vi "Server.vi"() -> ()   [LabVIEW 2019]
uses:
  padrao_todos_os_dados_ENTRADA.ctl
  padrao_UCM.004.EEL.0300_ENTRADA.ctl
  padrao_UCM.004.EEL.0200_ENTRADA.ctl
  padrao_INTERNO.ctl
  padrao_todos_os_dados_SAIDA.ctl
  padrao_UCM.004.EEL.0300_SAIDA.ctl
  padrao_UCM.004.EEL.0200_SAIDA.ctl
  padrao_tipo_dado.ctl
  padrao_enum.ctl
  padrao_dados_cliente_para_server.ctl
  padrao_informacoes_meu_computador.ctl
  padrao_TAGS_prioridades_client.ctl
panel:
  in  "Help Button":bool
  in  "Abrir central de certificados":bool
  in  "Abre conversao e link":bool
  out "Array tipo de dado":T1[](array[typedef]) items=["Engenharia", "Puro(mA)"]
  in  "puro_todos_os_dados_ENTRADA":T2
  out "todos_dados_SAIDA":T6
  in  "engenharia_todos_os_dados_ENTRADA":T2
  in  "Editor Vinculos":bool
  in  "Calibração":bool
  in  "Closed":refnum<k5>
  out "IPs Conectados":string[](array[string])
  out "led_indica_server_ligado":bool
  out "status":string
  out "Clients Conectados":string[](array[string])
  out "Quantidade de Clients":i32
  out "Erro Nessa VI":errorcluster
  in  "[ESC]":bool
  # "SERVER"
  # "1)  Rode o Server antes de rodar os Clients\n2) Rode o Server: Aperte Ctrl+R ou rode na seta la em cima \n3) Verifique se o Led Acendeu:  Ele deve ficar laranja\n4) A cada Client ligado, ira aparecer na lista de clients\n5) Monitore a barra de status para saber o que está acontecendo\n6) Caso haja problema com troca de dados, utilize o debug ou monitore os dados.\n7) Para desligar o Server, desligue os Clients primeiro, quando a quantidade de Clients for igual a zero, aperte ESC ou no botão STOP."
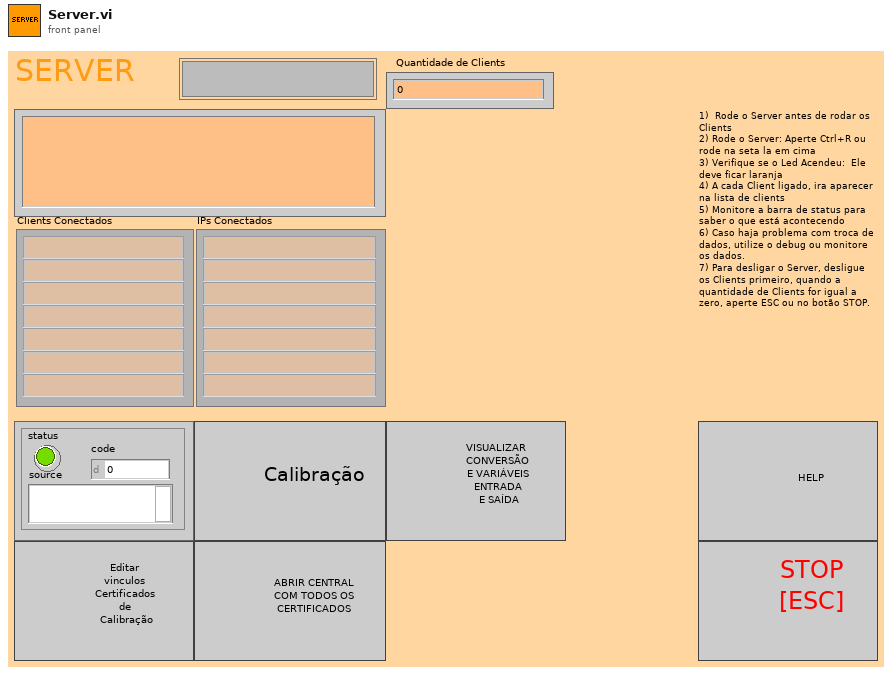
[diagram p1: front panel]
types:
  T1 = typedef "padrao_tipo_dado.ctl" = u16
  T2 = typedef "padrao_todos_os_dados_ENTRADA.ctl" = cluster{"UCM.004.EEL.0300_ENTRADA":T3, "UCM.004.EEL.0200_ENTRADA":T4, "INTERNO":T5}
  T3 = typedef "padrao_UCM.004.EEL.0300_ENTRADA.ctl" = cluster{"DIGITAL":cluster{"X30 1":bool, "X30 2":bool, "X30 3":bool, "X30 4":bool, "X30 5":bool, "X30 6":bool, "X30 7":bool, "X30 8":bool, "X30 9":bool, "X30 10":bool, "X30 11":bool, "X30 12":bool, "X30 13":bool, "X30 14":bool, "X30 15":bool, "X30 16":bool, "SPK-RD-ALR":bool, "SPK-RD-VVT":bool, "SPK-RD-FLL":bool, "SPW-RD-ALR":bool, "SPW-RD-VVT":bool, "SPW-RD-FLL":bool}, "ANALOGICO":cluster{"SKM-PA-BAR":i16, "SKM-PA-TQ":i16, "SKM-TI-TQ":i16, "SKM-PA-LAM":i16, "SKM-TI-LAM":i16, "SKM-PD-LAM":i16, "SKM-TI-WF":i16, "SKM-FIM-WF":i16, "SIT-PI-001":i16, "SKI-PD-ST":i16, "SIT-PI-MS1":i16, "SIT-PI-MS2":i16, "SKM-TI-KF":i16, "SPW-PD-P":i16, "SPK-PD-P":i16, "X32 16 ":i16, "X32 17":i16, "X32 18":i16, "X32 19":i16, "X32 20":i16, "X32 21":i16, "X32 22":i16, "X32 23":i16, "X32 24":i16, "SPK-RD-ST":i32, "SPW-RD-ST":i32, "SPK-RD-VEL":i32, "SPW-RD-VEL":i32, "SPK-RD-IA":i32, "SPW-RD-IA":i32, "SPK-RD-TU":i32, "SPW-RD-TU":i32, "SKM-TI-COR-KF":dbl, "SKM-DEN-COR-KF":dbl, "SKM-FIC-COR-KF":dbl, "SKM-TI-COR-AR":dbl, "SKM-DEN-COR-AR":dbl, "SPK-RD-CRT":dbl, "SPW-RD-CRT":dbl, "SKM-FIC-COR-AR":dbl}}
  T4 = typedef "padrao_UCM.004.EEL.0200_ENTRADA.ctl" = cluster{"DIGITAL":cluster{"SKS-LAH-S":bool, "SKS-LAH-W":bool, "SKS-LAH-K":bool, "SKS-MIN-W":bool, "SKS-MAX-W":bool, "SKS-MIN-K":bool, "SKS-MAX-K":bool, "X30-8":bool, "X30-9":bool, "X30-10":bool, "X30-11":bool, "X30-12":bool, "X30-13":bool, "X30-14":bool, "X30-15":bool, "X30-16":bool}, "ANALOGICO":cluster{"SKS-LC-K":i16, "SKS-LC-W":i16, "SHD-TI-AMB":i16, "X32-4":i16, "SHD-PI-01":i16, "SHD-PI-02":i16, "SIT-PI-MS3":i16, "SIT-PI-03":i16}}
  T5 = typedef "padrao_INTERNO.ctl" = cluster{"DIGITAL":cluster{"INTERNO-SI-SS-1":bool, "INTERNO-SI-SS-2":bool, "INTERNO-SI-SS-3":bool, "INTERNO-SS-SW-1":bool, "INTERNO-SS-SK-1":bool}, "ANALOGICO":cluster{"com_pc_analog":dbl}}
  T6 = typedef "padrao_todos_os_dados_SAIDA.ctl" = cluster{"UCM.004.EEL.0300_SAIDA":T7, "UCM.004.EEL.0200_SAIDA":T8, "INTERNO":T5}
  T7 = typedef "padrao_UCM.004.EEL.0300_SAIDA.ctl" = cluster{"DIGITAL":cluster{"SPK-CV-001":bool, "SPK-CV-002":bool, "SPK-CV-003":bool, "SPK-CV-004":bool, "SPK-CV-005":bool, "SPK-CV-006":bool, "SPK-CV-007":bool, "SPK-CV-008":bool, "SPW-CV-001":bool, "SPW-CV-002":bool, "SPW-CV-003":bool, "SPW-CV-004":bool, "SPW-CV-005":bool, "SPW-CV-006":bool, "SPW-CV-007":bool, "SPW-CV-008":bool, "SKM-CV-LAM":bool, "SKM-CV-COR":bool, "SKM-CV-JMP":bool, "SKI-CV-AR":bool, "SKI-CV-KF-ST":bool, "SKI-CV-KF-BY1":bool, "SKI-CV-WF-ST":bool, "SKI-CV-WF-BY1":bool, "SKI-CV-ST":bool, "SKI-CV-BY2":bool, "X31-27":bool, "X31-28":bool, "X31-29":bool, "X31-30":bool, "X31-31":bool, "X31-32":bool, "PID-PC-TQ-ON":bool, "PID-FC-AR-ON":bool, "PID-WF-ON":bool, "PID-KF-ON":bool, "PID-SA-WF-INV":bool, "PID-SA-KF-INV":bool, "PID-SA-AR-COR":bool, "SPK-WR-ON":bool, "SPW-WR-ON":bool, "SPK-WR-OFF":bool, "SPW-WR-OFF":bool}, "ANALOGICO":cluster{"SKM-PC-TQ":i16, "SKM-FC-AR":i16, "SKM-FC-WF":i16, "SKM-FC-KF":i16, "X33 5":i16, "X33 6":i16, "X33 7":i16, "X33 8":i16, "X33 9":i16, "X33 10":i16, "X33 11":i16, "X33 12":i16, "X33 13":i16, "X33 14":i16, "PID-PC-TQ-SP":i16, "PID-FC-AR-SP":i16, "PID-FC-WF-SP":i16, "PID-FC-KF-SP":i16, "PID-INC-WF-SP":i16, "PID-INC-KF-SP":i16, "SPK-WR-VEL":i32, "SPW-WR-VEL":i32, "SKM-FIC-COR-AR-MAX":dbl, "SKM-FIC-COR-AR-MIN":dbl, "SKM-FIC-COR-KF-MAX":dbl, "SKM-FIC-COR-KF-MIN":dbl, "PID-PC-TQ-GP":dbl, "PID-PC-TQ-GI":dbl, "PID-PC-TQ-GD":dbl, "PID-FC-AR-GP":dbl, "PID-FC-AR-GI":dbl, "PID-FC-AR-GD":dbl, "PID-FC-WF-GP":dbl, "PID-FC-WF-GI":dbl, "PID-FC-WF-GD":dbl, "PID-FC-KF-GP":dbl, "PID-FC-KF-GI":dbl, "PID-FC-KF-GD":dbl, "PID-INV-WF-GP":dbl, "PID-INV-WF-GI":dbl, "PID-INV-WF-GD":dbl, "PID-INV-KF-GP":dbl, "PID-INV-KF-GI":dbl, "PID-INV-KF-GD":dbl}}
  T8 = typedef "padrao_UCM.004.EEL.0200_SAIDA.ctl" = cluster{"DIGITAL":cluster{"SKS-CV-001":bool, "SKS-CV-002":bool, "SKS-CV-003":bool, "SKS-CV-004":bool, "SKS-CV-005":bool, "SKS-CV-006":bool, "SHD-CV-001":bool, "SHD-CV-002":bool, "SHD-ON-OFF":bool, "X31-10":bool, "X31-11":bool, "X31-12":bool, "X31-13":bool, "X31-14":bool, "X31-15":bool, "X31-16":bool}, "ANALOGICO":cluster{"GD-ST-ES":i16, "X33-2":i16}}
  T9 = typedef "padrao_enum.ctl" = enum16{"open-conection ", "data", "check-status", "Inicio"}
  T10 = enum32{"Invalid", "Standard", "Closed", "Hidden", "Minimized", "Maximized"}
  T11 = typedef "padrao_dados_cliente_para_server.ctl" = cluster{"todos_os_dados_saida":T6, "informacoes_meu_PC":T12, "padrao_prioridade_TAGs":T13}
  T12 = typedef "padrao_informacoes_meu_computador.ctl" = cluster{"Nome_computador":string, "IP_meu_computador":string, "Tipo de Dado":T1}
  T13 = typedef "padrao_TAGS_prioridades_client.ctl" = cluster{"TAG":string, "Tenho\nPrioridade?":bool}[]
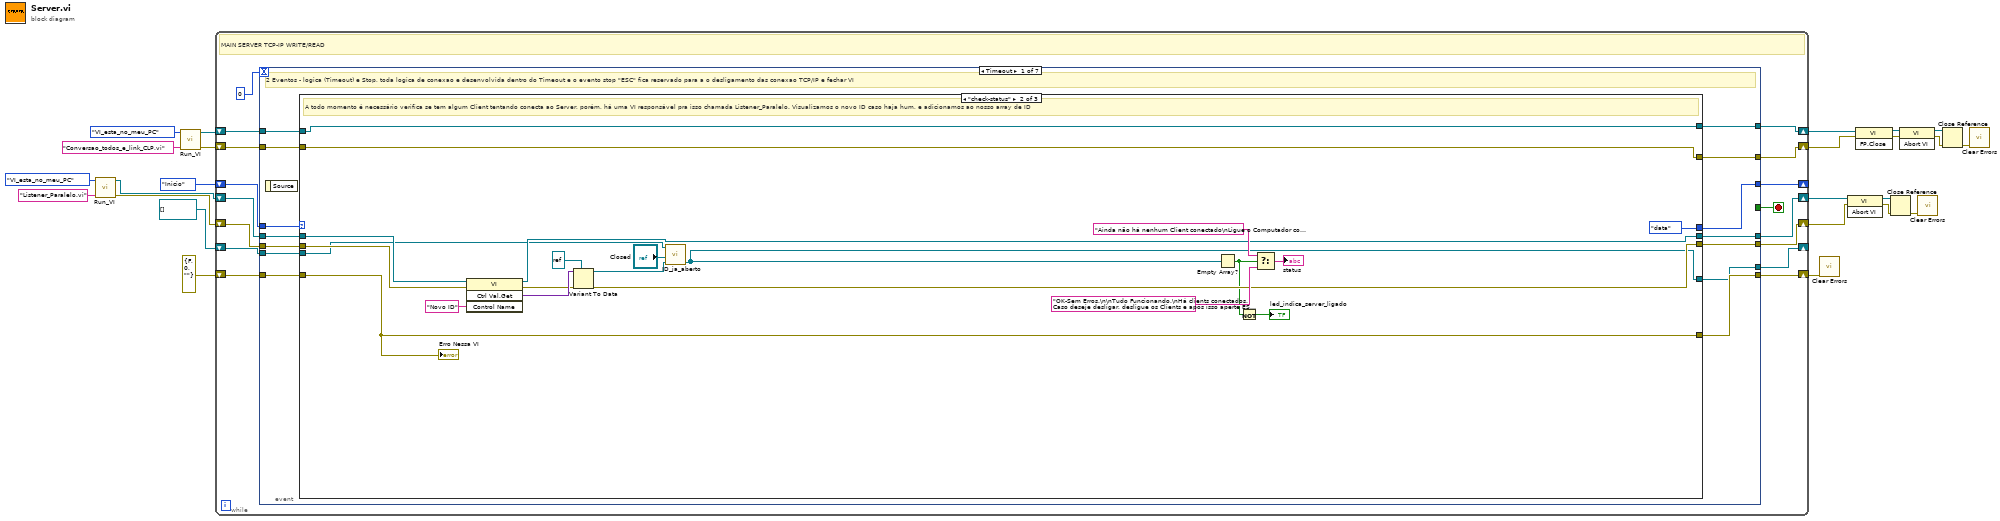
[diagram p0: block diagram]
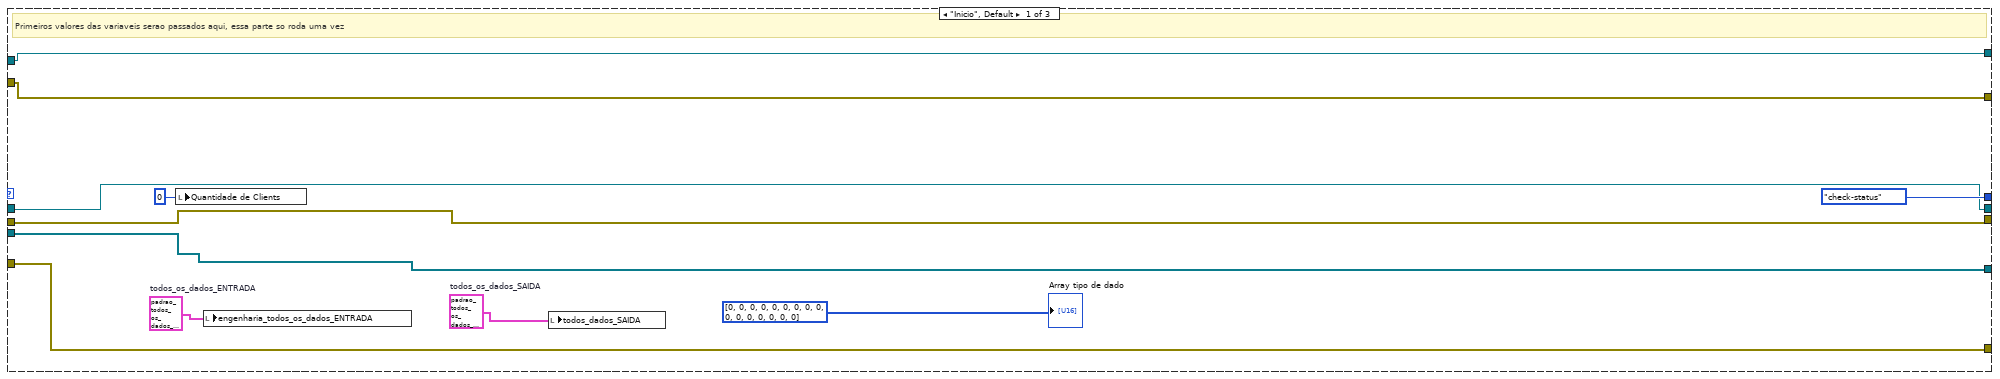
[diagram p2: hidden frame]
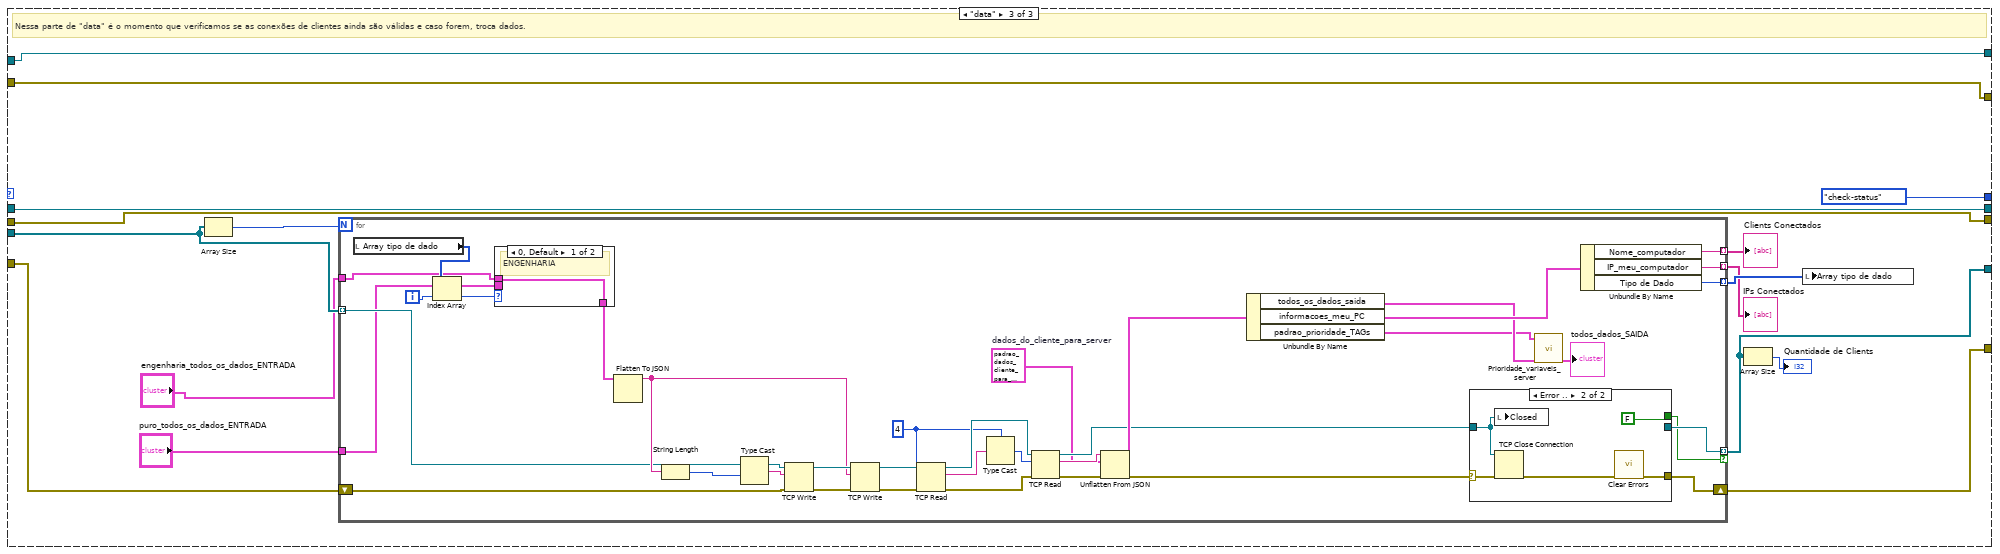
[diagram p3: hidden frame]
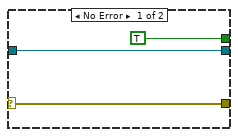
[diagram p5: hidden frame]
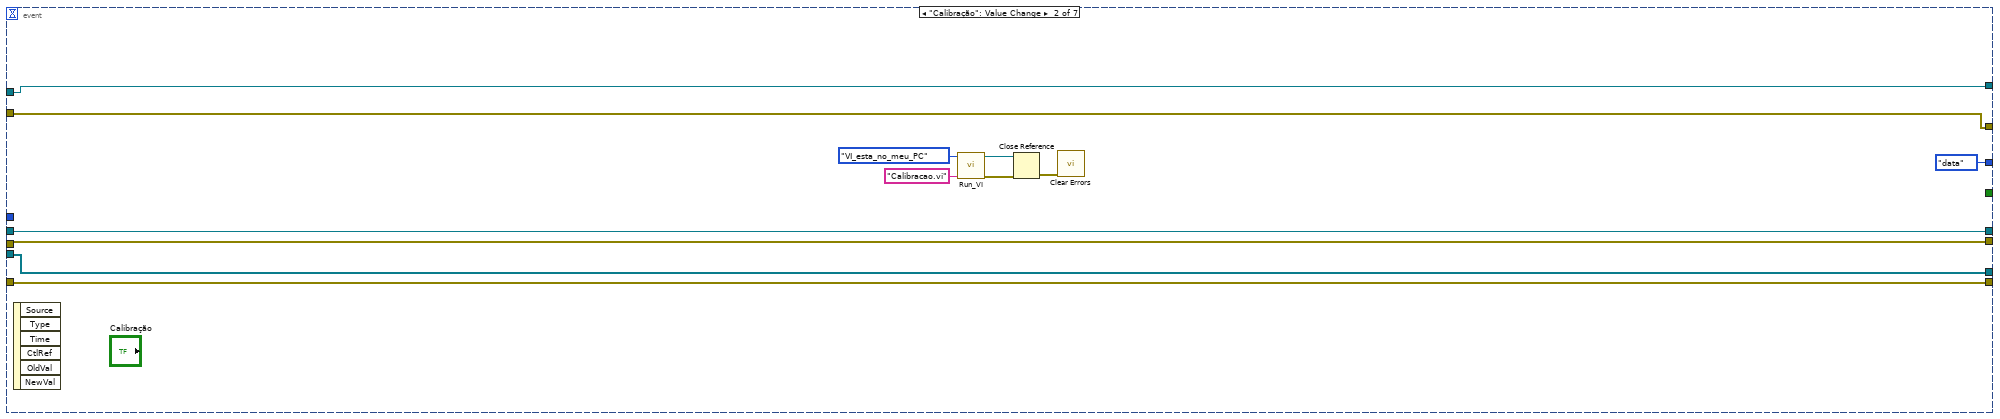
[diagram p6: hidden frame]
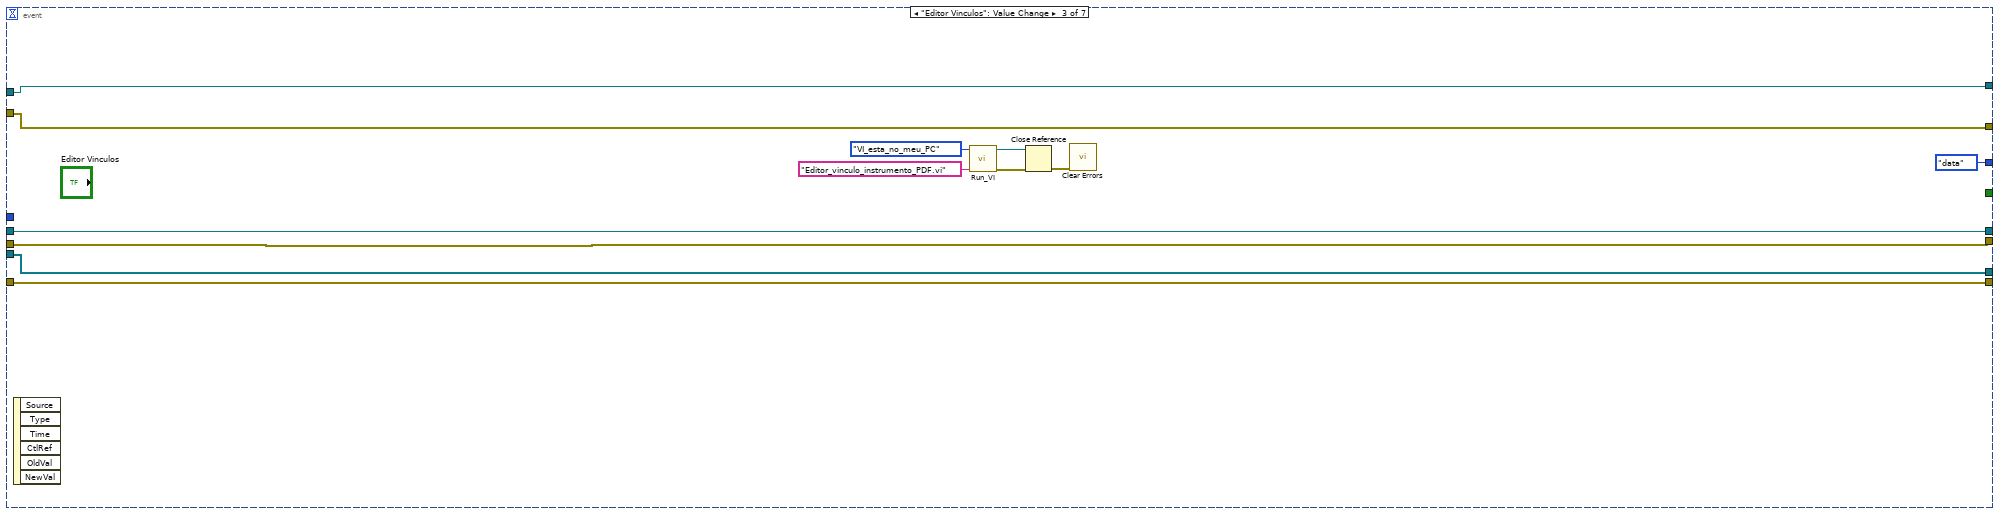
[diagram p7: hidden frame]
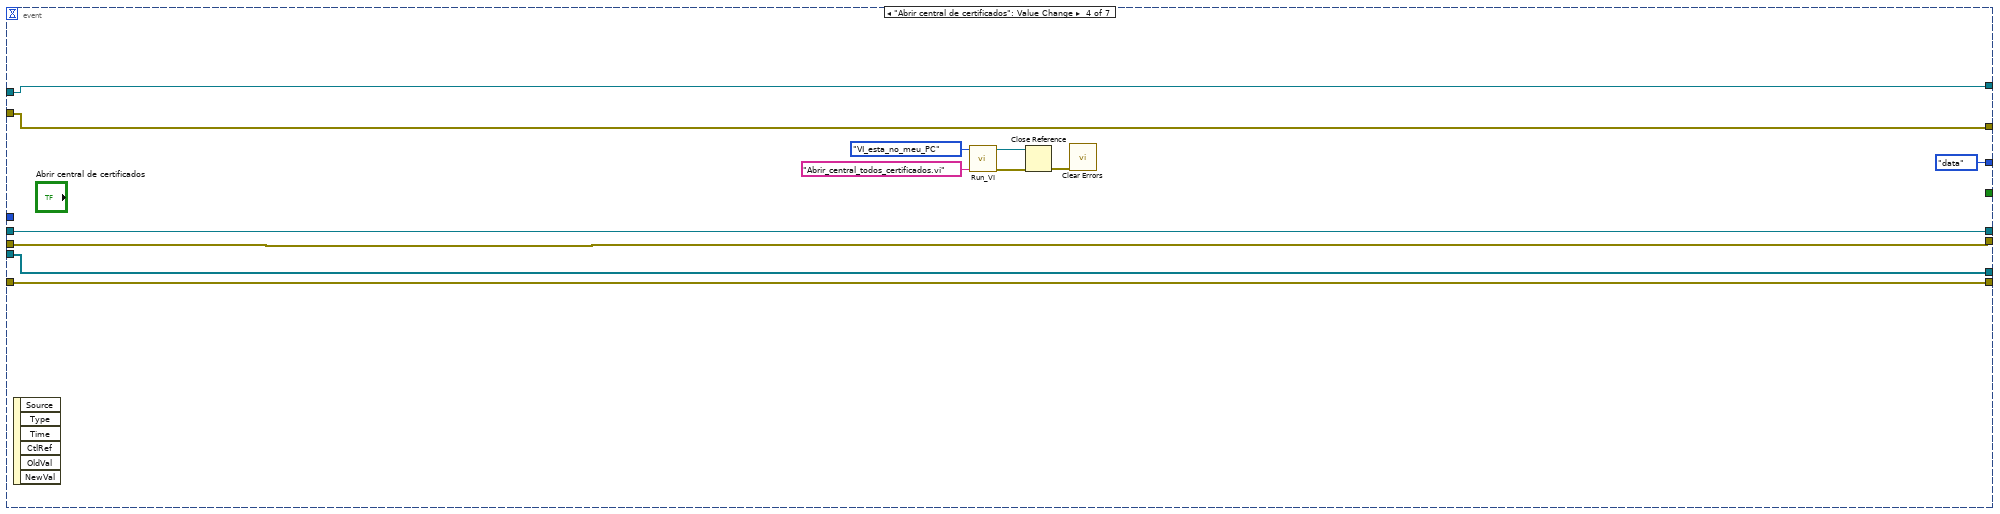
[diagram p8: hidden frame]
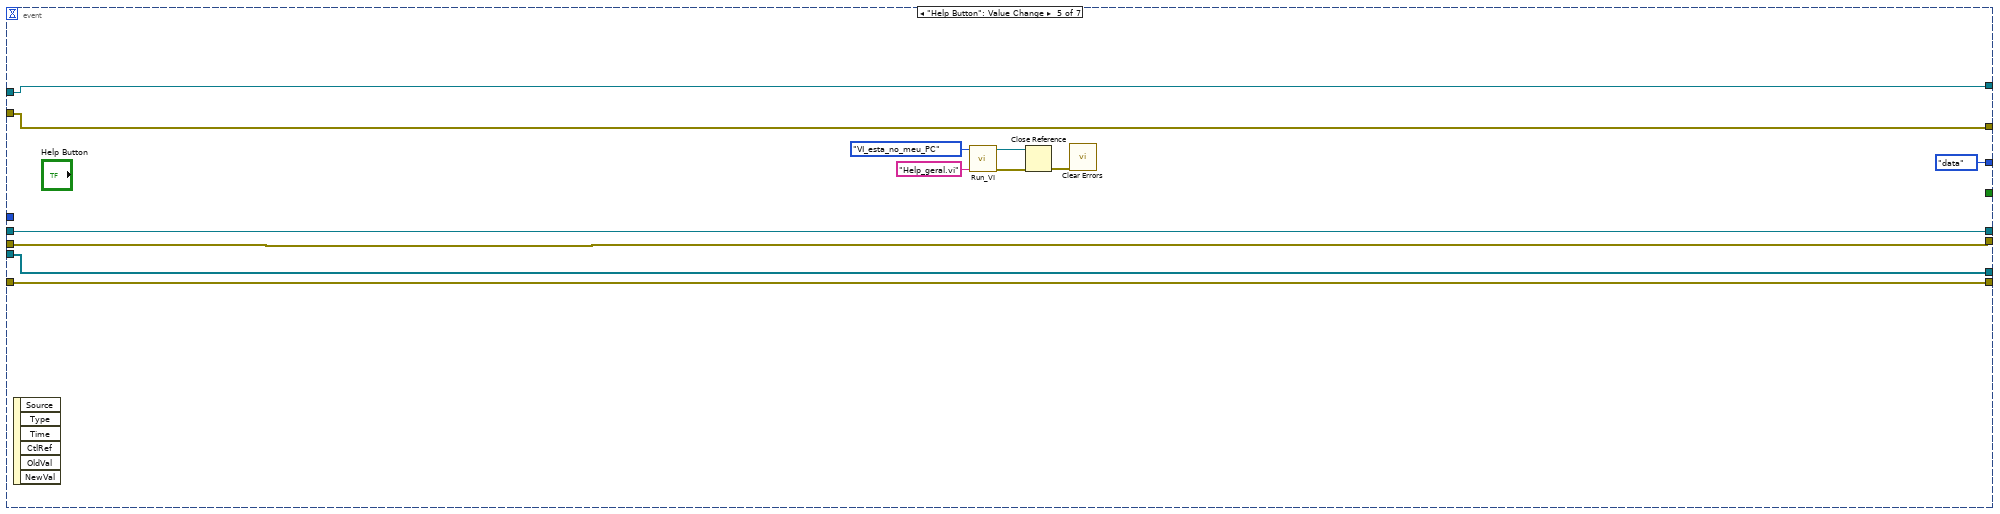
[diagram p9: hidden frame]
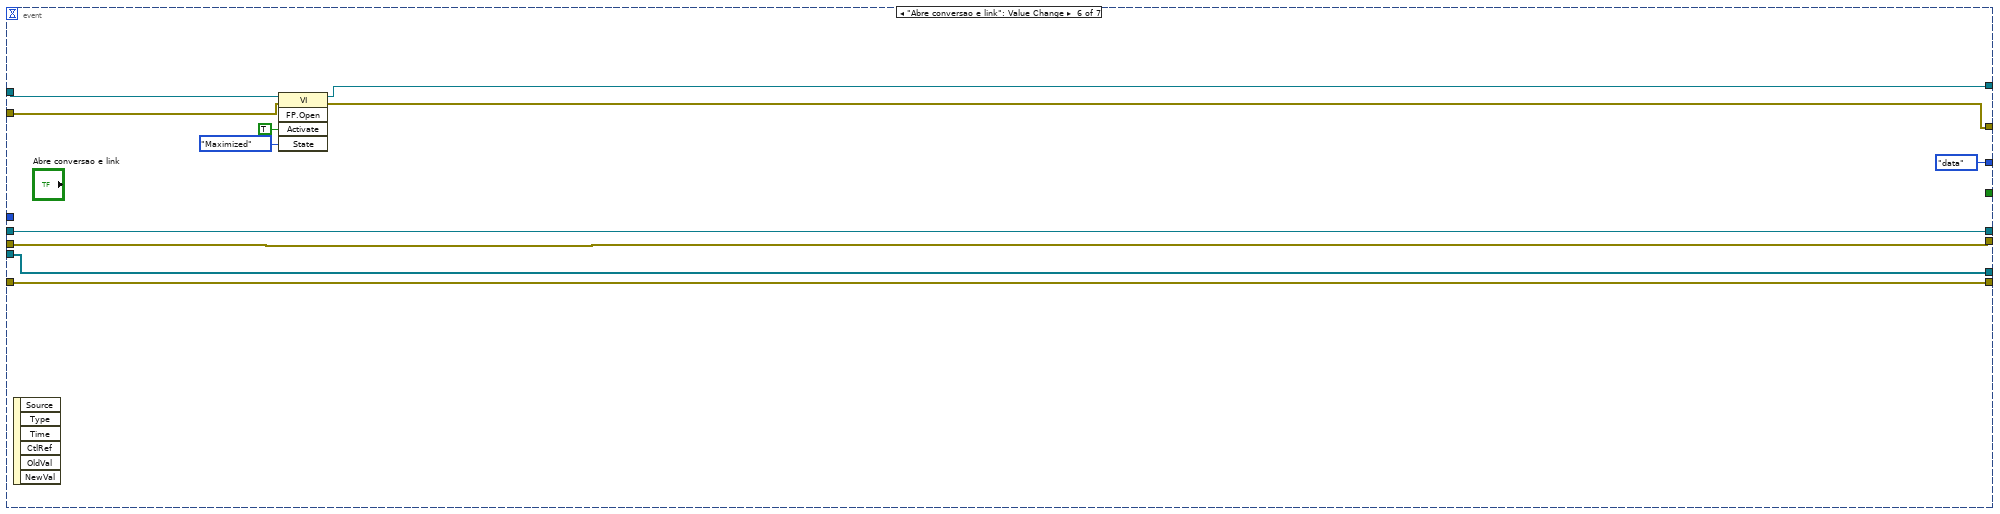
[diagram p10: hidden frame]
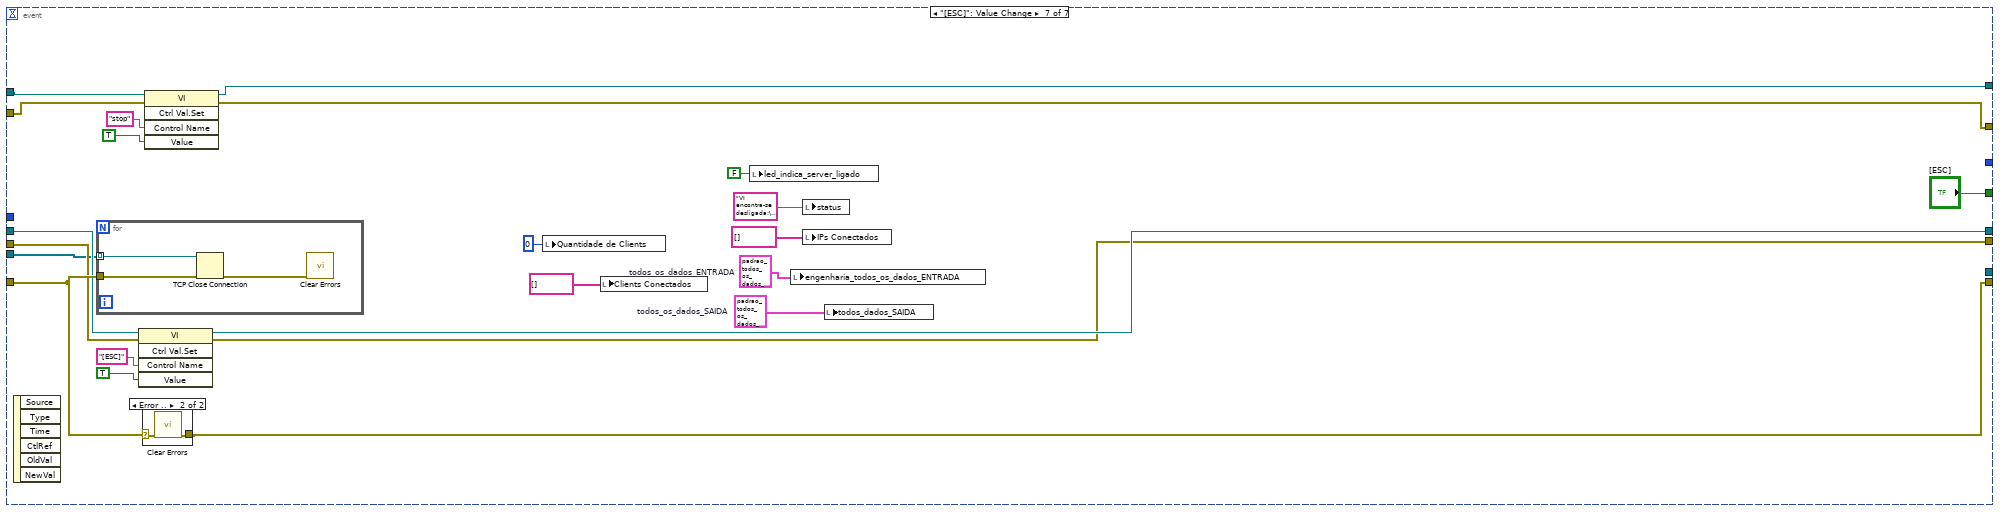
[diagram p11: hidden frame]
diagram:
  n1 = call "Run_VI.vi"("Nome.vi"="Listener_Paralelo.vi", "Origem_VI"=enum16{"VI_esta_no_meu_PC", "VI_esta_na_rede"}."VI_esta_no_meu_PC") -> ("error out"=w22:errorcluster, "reference out"=w21:refnum<vi>)  [unwired: 8 in]
  n2 = call "Run_VI.vi"("Nome.vi"="Conversao_todos_e_link_CLP.vi", "Origem_VI"=enum16{"VI_esta_no_meu_PC", "VI_esta_na_rede"}."VI_esta_no_meu_PC") -> ("error out"=w8:errorcluster, "reference out"=w9:refnum<vi>)  [unwired: 8 in]
  n3 = while {
    shift-right: [w34] -> _
    shift-left: padrao_enum."Inicio" ("Enum") -> [w39]
    shift-right: [w37] -> w13
    shift-left: errorcluster {"status"=FALSE, "code"=0, "source"=""} ("error constant") -> [w38]
    shift-right: [w33] -> _
    shift-left: refnum<k5>[] [] ("appended array") -> [w36]
    shift-right: [w30] -> w19
    shift-left: w21 -> [w32]
    shift-right: [w29] -> w18
    shift-left: w22 -> [w31]
    shift-right: [w26] -> w4
    shift-left: w9 -> [w28]
    shift-right: [w25] -> w3
    shift-left: w8 -> [w27]
    stop <- w40 stop-if-true
    # "MAIN SERVER TCP-IP WRITE/READ"
    n4 = event shown="[0] Timeout" {
      selector: _ -> [_ _ _ _ _ _ _]
      dyn-events: _ -> [_ _ _ _ _ _ _]
      timeout: 0 -> [_ _ _ _ _ _ _]
      tunnel: [_ _ _ _ _ _ "[ESC]"] -> w40
      tunnel: w39 -> [w51 _ _ _ _ _ _]
      tunnel: w38 -> [w54 w149 w161 w173 w185 w203 w228]
      tunnel: [w53 w149 w161 w173 w185 w203 w229] -> w37
      tunnel: w36 -> [w52 w150 w162 w174 w186 w204 w219]
      tunnel: [w50 padrao_enum."data" ("Enum") padrao_enum."data" ("Enum") padrao_enum."data" ("Enum") padrao_enum."data" ("Enum") padrao_enum."data" ("Enum") _] -> w34
      tunnel: [w49 w150 w162 w174 w186 w204 _] -> w33
      tunnel: w32 -> [w48 w152 w164 w176 w188 w206 w225]
      tunnel: w31 -> [w47 w151 w163 w175 w187 w205 w224]
      tunnel: [w46 w152 w164 w176 w188 w206 w221] -> w30
      tunnel: [w45 w151 w163 w175 w187 w205 w220] -> w29
      tunnel: w28 -> [w44 w154 w167 w179 w191 w202 w211]
      tunnel: w27 -> [w43 w153 w166 w178 w190 w201 w210]
      tunnel: [w42 w154 w167 w179 w191 w199 w209] -> w26
      tunnel: [w41 w153 w166 w178 w190 w198 w208] -> w25
      event Timeout {
        # "2 Eventos - logica (Timeout) e Stop, toda logica de conexao e desenvolvida dentro do Timeout e o evento stop \"ESC\" fica reservado para a o desligamento das conexao TCP/IP e fechar VI"
        n5 = event-data() -> ()  [unwired: 1 in, 1 out]
        n6 = case shown="\"check-status\"" w51 {
          tunnel: w54 -> [w64 w83 w101]
          tunnel: [w64 w83 w100] -> w53
          tunnel: w52 -> [w63 w73 w95]
          tunnel: [padrao_enum."check-status" ("Enum") padrao_enum."data" ("Enum") padrao_enum."check-status" ("Enum")] -> w50
          tunnel: [w63 w70 w94] -> w49
          tunnel: w48 -> [w61 w77 w99]
          tunnel: w47 -> [w60 w76 w98]
          tunnel: [w61 w75 w99] -> w46
          tunnel: [w60 w74 w98] -> w45
          tunnel: w44 -> [w57 w67 w88]
          tunnel: w43 -> [w56 w66 w87]
          tunnel: [w57 w67 w88] -> w42
          tunnel: [w56 w66 w87] -> w41
          frame "Inicio", Default {
            w58 = T6 {"UCM.004.EEL.0300_SAIDA"={"DIGITAL"={"SPK-CV-001"=FALSE, "SPK-CV-002"=FALSE, "SPK-CV-003"=FALSE, "SPK-CV-004"=FALSE, "SPK-CV-005"=FALSE, "SPK-CV-006"=FALSE, "SPK-CV-007"=FALSE, "SPK-CV-008"=FALSE, "SPW-CV-001"=FALSE, "SPW-CV-002"=FALSE, "SPW-CV-003"=FALSE, "SPW-CV-004"=FALSE, "SPW-CV-005"=FALSE, "SPW-CV-006"=FALSE, "SPW-CV-007"=FALSE, "SPW-CV-008"=FALSE, "SKM-CV-LAM"=FALSE, "SKM-CV-COR"=FALSE, "SKM-CV-JMP"=FALSE, "SKI-CV-AR"=FALSE, "SKI-CV-KF-ST"=FALSE, "SKI-CV-KF-BY1"=FALSE, "SKI-CV-WF-ST"=FALSE, "SKI-CV-WF-BY1"=FALSE, "SKI-CV-ST"=FALSE, "SKI-CV-BY2"=FALSE, "X31-27"=FALSE, "X31-28"=FALSE, "X31-29"=FALSE, "X31-30"=FALSE, "X31-31"=FALSE, "X31-32"=FALSE, "PID-PC-TQ-ON"=FALSE, "PID-FC-AR-ON"=FALSE, "PID-WF-ON"=FALSE, "PID-KF-ON"=FALSE, "PID-SA-WF-INV"=FALSE, "PID-SA-KF-INV"=FALSE, "PID-SA-AR-COR"=FALSE, "SPK-WR-ON"=FALSE, "SPW-WR-ON"=FALSE, "SPK-WR-OFF"=FALSE, "SPW-WR-OFF"=FALSE}, "ANALOGICO"={"SKM-PC-TQ"=0, "SKM-FC-AR"=0, "SKM-FC-WF"=0, "SKM-FC-KF"=0, "X33 5"=0, "X33 6"=0, "X33 7"=0, "X33 8"=0, "X33 9"=0, "X33 10"=0, "X33 11"=0, "X33 12"=0, "X33 13"=0, "X33 14"=0, "PID-PC-TQ-SP"=0, "PID-FC-AR-SP"=0, "PID-FC-WF-SP"=0, "PID-FC-KF-SP"=0, "PID-INC-WF-SP"=0, "PID-INC-KF-SP"=0, "SPK-WR-VEL"=0, "SPW-WR-VEL"=0, "SKM-FIC-COR-AR-MAX"=0.0, "SKM-FIC-COR-AR-MIN"=0.0, "SKM-FIC-COR-KF-MAX"=0.0, "SKM-FIC-COR-KF-MIN"=0.0, "PID-PC-TQ-GP"=0.0, "PID-PC-TQ-GI"=0.0, "PID-PC-TQ-GD"=0.0, "PID-FC-AR-GP"=0.0, "PID-FC-AR-GI"=0.0, "PID-FC-AR-GD"=0.0, "PID-FC-WF-GP"=0.0, "PID-FC-WF-GI"=0.0, "PID-FC-WF-GD"=0.0, "PID-FC-KF-GP"=0.0, "PID-FC-KF-GI"=0.0, "PID-FC-KF-GD"=0.0, "PID-INV-WF-GP"=0.0, "PID-INV-WF-GI"=0.0, "PID-INV-WF-GD"=0.0, "PID-INV-KF-GP"=0.0, "PID-INV-KF-GI"=0.0, "PID-INV-KF-GD"=0.0}}, "UCM.004.EEL.0200_SAIDA"={"DIGITAL"={"SKS-CV-001"=FALSE, "SKS-CV-002"=FALSE, "SKS-CV-003"=FALSE, "SKS-CV-004"=FALSE, "SKS-CV-005"=FALSE, "SKS-CV-006"=FALSE, "SHD-CV-001"=FALSE, "SHD-CV-002"=FALSE, "SHD-ON-OFF"=FALSE, "X31-10"=FALSE, "X31-11"=FALSE, "X31-12"=FALSE, "X31-13"=FALSE, "X31-14"=FALSE, "X31-15"=FALSE, "X31-16"=FALSE}, "ANALOGICO"={"GD-ST-ES"=0, "X33-2"=0}}, "INTERNO"={"DIGITAL"={"INTERNO-SI-SS-1"=FALSE, "INTERNO-SI-SS-2"=FALSE, "INTERNO-SI-SS-3"=FALSE, "INTERNO-SS-SW-1"=FALSE, "INTERNO-SS-SK-1"=FALSE}, "ANALOGICO"={"com_pc_analog"=0.0}}}  # todos_os_dados_SAIDA
            w59 = T2 {"UCM.004.EEL.0300_ENTRADA"={"DIGITAL"={"X30 1"=FALSE, "X30 2"=FALSE, "X30 3"=FALSE, "X30 4"=FALSE, "X30 5"=FALSE, "X30 6"=FALSE, "X30 7"=FALSE, "X30 8"=FALSE, "X30 9"=FALSE, "X30 10"=FALSE, "X30 11"=FALSE, "X30 12"=FALSE, "X30 13"=FALSE, "X30 14"=FALSE, "X30 15"=FALSE, "X30 16"=FALSE, "SPK-RD-ALR"=FALSE, "SPK-RD-VVT"=FALSE, "SPK-RD-FLL"=FALSE, "SPW-RD-ALR"=FALSE, "SPW-RD-VVT"=FALSE, "SPW-RD-FLL"=FALSE}, "ANALOGICO"={"SKM-PA-BAR"=0, "SKM-PA-TQ"=0, "SKM-TI-TQ"=0, "SKM-PA-LAM"=0, "SKM-TI-LAM"=0, "SKM-PD-LAM"=0, "SKM-TI-WF"=0, "SKM-FIM-WF"=0, "SIT-PI-001"=0, "SKI-PD-ST"=0, "SIT-PI-MS1"=0, "SIT-PI-MS2"=0, "SKM-TI-KF"=0, "SPW-PD-P"=0, "SPK-PD-P"=0, "X32 16 "=0, "X32 17"=0, "X32 18"=0, "X32 19"=0, "X32 20"=0, "X32 21"=0, "X32 22"=0, "X32 23"=0, "X32 24"=0, "SPK-RD-ST"=0, "SPW-RD-ST"=0, "SPK-RD-VEL"=0, "SPW-RD-VEL"=0, "SPK-RD-IA"=0, "SPW-RD-IA"=0, "SPK-RD-TU"=0, "SPW-RD-TU"=0, "SKM-TI-COR-KF"=0.0, "SKM-DEN-COR-KF"=0.0, "SKM-FIC-COR-KF"=0.0, "SKM-TI-COR-AR"=0.0, "SKM-DEN-COR-AR"=0.0, "SPK-RD-CRT"=0.0, "SPW-RD-CRT"=0.0, "SKM-FIC-COR-AR"=0.0}}, "UCM.004.EEL.0200_ENTRADA"={"DIGITAL"={"SKS-LAH-S"=FALSE, "SKS-LAH-W"=FALSE, "SKS-LAH-K"=FALSE, "SKS-MIN-W"=FALSE, "SKS-MAX-W"=FALSE, "SKS-MIN-K"=FALSE, "SKS-MAX-K"=FALSE, "X30-8"=FALSE, "X30-9"=FALSE, "X30-10"=FALSE, "X30-11"=FALSE, "X30-12"=FALSE, "X30-13"=FALSE, "X30-14"=FALSE, "X30-15"=FALSE, "X30-16"=FALSE}, "ANALOGICO"={"SKS-LC-K"=0, "SKS-LC-W"=0, "SHD-TI-AMB"=0, "X32-4"=0, "SHD-PI-01"=0, "SHD-PI-02"=0, "SIT-PI-MS3"=0, "SIT-PI-03"=0}}, "INTERNO"={"DIGITAL"={"INTERNO-SI-SS-1"=FALSE, "INTERNO-SI-SS-2"=FALSE, "INTERNO-SI-SS-3"=FALSE, "INTERNO-SS-SW-1"=FALSE, "INTERNO-SS-SK-1"=FALSE}, "ANALOGICO"={"com_pc_analog"=0.0}}}  # todos_os_dados_ENTRADA
            w55 = T1[] [0, 0, 0, 0, 0, 0, 0, 0, 0, 0, 0, 0, 0, 0, 0, 0] items=["Engenharia", "Puro(mA)"] ("Array")
            # "Primeiros valores das variaveis serao passados aqui, essa parte so roda uma vez"
            n7 = local write "Quantidade de Clients"(0 ("size(s)")) -> ()
            n8 = local write "engenharia_todos_os_dados_ENTRADA"(w59) -> ()
            n9 = local write "todos_dados_SAIDA"(w58) -> ()
            "Array tipo de dado" <- w55
          }
          frame "check-status" {
            # "A todo momento é necessário verifica se tem algum Client tentando conecta ao Server, porém, há uma VI responsável pra isso chamada Listener_Paralelo. Visualizamos o novo ID caso haja hum, e adicionamos ao nosso array de ID"
            n10 = invoke class="VI" method="Ctrl Val.Get"(reference=w77, error in=w76, "Control Name"="Novo ID") -> (reference out=w75:refnum<vi>, error out=w78:errorcluster, "Get Control Value Variant"=w80:variant)  [unwired: 1 in, 1 out]
            n11 = Variant To Data(error in=w78, type=refnum<k5> refnum ("listener ID"), Variant=w80) -> (data=w71:refnum<k5>, error out=w74:errorcluster)
            n12 = call "ID_ja_aberto.vi"("Conexao nova"=w71, "Conexao fechada"="Closed", "Entrada Array Conexao"=w73) -> ("Saida Array Conexao"=w70:refnum<k5>[])  [unwired: 8 in]
            n13 = Empty Array?(array=w70) -> (empty?=w68:bool)
            n14 = Not(x=w68) -> (.not. x?=→"led_indica_server_ligado":bool)
            n15 = Select(t="Ainda não há nenhum Client conectado\nLigue o Computador com o Client que deseje utilizar\nAperte ESC caso deseje encerrar", s=w68, f="OK-Sem Erros.\n\nTudo Funcionando.\nHá clients conectados. Caso deseje desligar, desligue os Clients e após isso aperte ESC nessa VI") -> (s? t:f=→"status":string)
            "Erro Nessa VI" <- w83
          }
          frame "data" {
            # "Nessa parte de \"data\" é o momento que verificamos se as conexões de clientes ainda são válidas e caso forem, troca dados."
            n16 = Array Size(array=w95) -> (size(s)=w96:i32)
            n17 = for {
              N: w96 -> [_]
              tunnel: w95 -> [w132] mode=indexing
              shift-right: [w116] -> w100
              shift-left: w101 -> [w138]
              tunnel: [w118] -> w94 mode=indexing if=w117
              tunnel: [w121] -> w91 mode=indexing
              tunnel: [w120] -> w93 mode=indexing
              tunnel: [w119] -> w92 mode=indexing
              tunnel: "engenharia_todos_os_dados_ENTRADA" -> [w107]
              tunnel: "puro_todos_os_dados_ENTRADA" -> [w106]
              i -> [w112]
              w104 = T11 {"todos_os_dados_saida"={"UCM.004.EEL.0300_SAIDA"={"DIGITAL"={"SPK-CV-001"=FALSE, "SPK-CV-002"=FALSE, "SPK-CV-003"=FALSE, "SPK-CV-004"=FALSE, "SPK-CV-005"=FALSE, "SPK-CV-006"=FALSE, "SPK-CV-007"=FALSE, "SPK-CV-008"=FALSE, "SPW-CV-001"=FALSE, "SPW-CV-002"=FALSE, "SPW-CV-003"=FALSE, "SPW-CV-004"=FALSE, "SPW-CV-005"=FALSE, "SPW-CV-006"=FALSE, "SPW-CV-007"=FALSE, "SPW-CV-008"=FALSE, "SKM-CV-LAM"=FALSE, "SKM-CV-COR"=FALSE, "SKM-CV-JMP"=FALSE, "SKI-CV-AR"=FALSE, "SKI-CV-KF-ST"=FALSE, "SKI-CV-KF-BY1"=FALSE, "SKI-CV-WF-ST"=FALSE, "SKI-CV-WF-BY1"=FALSE, "SKI-CV-ST"=FALSE, "SKI-CV-BY2"=FALSE, "X31-27"=FALSE, "X31-28"=FALSE, "X31-29"=FALSE, "X31-30"=FALSE, "X31-31"=FALSE, "X31-32"=FALSE, "PID-PC-TQ-ON"=FALSE, "PID-FC-AR-ON"=FALSE, "PID-WF-ON"=FALSE, "PID-KF-ON"=FALSE, "PID-SA-WF-INV"=FALSE, "PID-SA-KF-INV"=FALSE, "PID-SA-AR-COR"=FALSE, "SPK-WR-ON"=FALSE, "SPW-WR-ON"=FALSE, "SPK-WR-OFF"=FALSE, "SPW-WR-OFF"=FALSE}, "ANALOGICO"={"SKM-PC-TQ"=0, "SKM-FC-AR"=0, "SKM-FC-WF"=0, "SKM-FC-KF"=0, "X33 5"=0, "X33 6"=0, "X33 7"=0, "X33 8"=0, "X33 9"=0, "X33 10"=0, "X33 11"=0, "X33 12"=0, "X33 13"=0, "X33 14"=0, "PID-PC-TQ-SP"=0, "PID-FC-AR-SP"=0, "PID-FC-WF-SP"=0, "PID-FC-KF-SP"=0, "PID-INC-WF-SP"=0, "PID-INC-KF-SP"=0, "SPK-WR-VEL"=0, "SPW-WR-VEL"=0, "SKM-FIC-COR-AR-MAX"=0.0, "SKM-FIC-COR-AR-MIN"=0.0, "SKM-FIC-COR-KF-MAX"=0.0, "SKM-FIC-COR-KF-MIN"=0.0, "PID-PC-TQ-GP"=0.0, "PID-PC-TQ-GI"=0.0, "PID-PC-TQ-GD"=0.0, "PID-FC-AR-GP"=0.0, "PID-FC-AR-GI"=0.0, "PID-FC-AR-GD"=0.0, "PID-FC-WF-GP"=0.0, "PID-FC-WF-GI"=0.0, "PID-FC-WF-GD"=0.0, "PID-FC-KF-GP"=0.0, "PID-FC-KF-GI"=0.0, "PID-FC-KF-GD"=0.0, "PID-INV-WF-GP"=0.0, "PID-INV-WF-GI"=0.0, "PID-INV-WF-GD"=0.0, "PID-INV-KF-GP"=0.0, "PID-INV-KF-GI"=0.0, "PID-INV-KF-GD"=0.0}}, "UCM.004.EEL.0200_SAIDA"={"DIGITAL"={"SKS-CV-001"=FALSE, "SKS-CV-002"=FALSE, "SKS-CV-003"=FALSE, "SKS-CV-004"=FALSE, "SKS-CV-005"=FALSE, "SKS-CV-006"=FALSE, "SHD-CV-001"=FALSE, "SHD-CV-002"=FALSE, "SHD-ON-OFF"=FALSE, "X31-10"=FALSE, "X31-11"=FALSE, "X31-12"=FALSE, "X31-13"=FALSE, "X31-14"=FALSE, "X31-15"=FALSE, "X31-16"=FALSE}, "ANALOGICO"={"GD-ST-ES"=0, "X33-2"=0}}, "INTERNO"={"DIGITAL"={"INTERNO-SI-SS-1"=FALSE, "INTERNO-SI-SS-2"=FALSE, "INTERNO-SI-SS-3"=FALSE, "INTERNO-SS-SW-1"=FALSE, "INTERNO-SS-SK-1"=FALSE}, "ANALOGICO"={"com_pc_analog"=0.0}}}, "informacoes_meu_PC"={"Nome_computador"="", "IP_meu_computador"="", "Tipo de Dado"=0}, "padrao_prioridade_TAGs"=[]}  # dados_do_cliente_para_server
              w125 = 4 ("bytes to read")
              n18 = local read "Array tipo de dado"() -> (w113:T1[])
              n19 = Index Array(array=w113, index=w112) -> (element=w108:T1)
              n20 = case shown="0, Default" w108 {
                tunnel: w107 -> [w139 _]
                tunnel: w106 -> [_ w140]
                tunnel: [w139 w140] -> w105
                frame 0, Default {
                  # "ENGENHARIA"
                }
                frame 1 {
                  # "PURO"
                }
              }
              n21 = Flatten To JSON(anything=w105) -> (JSON string=w133:string)  [unwired: 2 in, 1 out]
              n22 = String Length(string=w133) -> (length=w135:i32)
              n23 = Type Cast(x=w135) -> (*(type *) &x=w134:string)  [unwired: 1 in]
              n24 = TCP Write(connection ID=w132, data in=w134, error in (no error)=w138) -> (connection ID out=w136:refnum<k5>, error out=w137:errorcluster)  [unwired: 2 out]
              n25 = TCP Write(connection ID=w136, data in=w133, error in (no error)=w137) -> (connection ID out=w131:refnum<k5>, error out=w130:errorcluster)  [unwired: 2 out]
              n26 = TCP Read(connection ID=w131, bytes to read=w125, error in (no error)=w130) -> (connection ID out=w129:refnum<k5>, data out=w126:string, error out=w128:errorcluster)  [unwired: 2 in]
              n27 = Type Cast(type=w125, x=w126) -> (*(type *) &x=w124:i32)
              n28 = TCP Read(connection ID=w129, bytes to read=w124, error in (no error)=w128) -> (connection ID out=w115:refnum<k5>, data out=w123:string, error out=w127:errorcluster)  [unwired: 2 in]
              n29 = Unflatten From JSON(JSON string=w123, type and defaults=w104, error in (no error)=w127) -> (value=w122:T11, error out=w114:errorcluster)  [unwired: 4 in]
              n30 = Unbundle By Name(w122) -> ("todos_os_dados_saida"=w110:T6, "informacoes_meu_PC"=w111:T12, "padrao_prioridade_TAGs"=w109:T13)
              n31 = case shown="Error .." w114 {
                selector: w114 -> [w143 w145]
                tunnel: w115 -> [w141 w144]
                tunnel: [w143 w148] -> w116
                tunnel: [TRUE FALSE] -> w117
                tunnel: [w141 _] -> w118
                frame No Error {
                }
                frame Error {
                  n32 = local write "Closed"(w144) -> ()
                  n33 = TCP Close Connection(connection ID=w144, error in (no error)=w145) -> (error out=w146:errorcluster)  [unwired: 1 in, 1 out]
                  n34 = call <vilib>:"Clear Errors.vi"("error in (no error)"=w146) -> ("error out"=w148:errorcluster)  [unwired: 5 in, 1 out]
                }
              }
              n35 = call "Prioridade_variaveis_server.vi"("dados_entrada_vindo_client"=w110, "padrao_TAGS_prioridade_client"=w109) -> ("dados_entrada_para_clp_priorizado"=→"todos_dados_SAIDA":T6)  [unwired: 9 in]
              n36 = Unbundle By Name(w111) -> ("Nome_computador"=w121:string, "IP_meu_computador"=w119:string, "Tipo de Dado"=w120:T1)
            }
            "Clients Conectados" <- w91
            "IPs Conectados" <- w92
            n37 = Array Size(array=w94) -> (size(s)=→"Quantidade de Clients":i32)
            n38 = local write "Array tipo de dado"(w93) -> ()
          }
        }
      }
      event "Calibração": Value Change {
        n39 = event-data() -> ()  [unwired: 1 in, 6 out]
        n40 = call "Run_VI.vi"("Nome.vi"="Calibracao.vi", "Origem_VI"=enum16{"VI_esta_no_meu_PC", "VI_esta_na_rede"}."VI_esta_no_meu_PC") -> ("error out"=w158:errorcluster, "reference out"=w159:refnum<vi>)  [unwired: 8 in]
        n41 = Close Reference(reference=w159, error in (no error)=w158) -> (error out=w157:errorcluster)
        n42 = call <vilib>:"Clear Errors.vi"("error in (no error)"=w157) -> ()  [unwired: 5 in, 2 out]
      }
      event "Editor Vinculos": Value Change {
        n43 = event-data() -> ()  [unwired: 1 in, 6 out]
        n44 = call "Run_VI.vi"("Nome.vi"="Editor_vinculo_instrumento_PDF.vi", "Origem_VI"=enum16{"VI_esta_no_meu_PC", "VI_esta_na_rede"}."VI_esta_no_meu_PC") -> ("error out"=w170:errorcluster, "reference out"=w171:refnum<vi>)  [unwired: 8 in]
        n45 = Close Reference(reference=w171, error in (no error)=w170) -> (error out=w169:errorcluster)
        n46 = call <vilib>:"Clear Errors.vi"("error in (no error)"=w169) -> ()  [unwired: 5 in, 2 out]
      }
      event "Abrir central de certificados": Value Change {
        n47 = event-data() -> ()  [unwired: 1 in, 6 out]
        n48 = call "Run_VI.vi"("Nome.vi"="Abrir_central_todos_certificados.vi", "Origem_VI"=enum16{"VI_esta_no_meu_PC", "VI_esta_na_rede"}."VI_esta_no_meu_PC") -> ("error out"=w182:errorcluster, "reference out"=w183:refnum<vi>)  [unwired: 8 in]
        n49 = Close Reference(reference=w183, error in (no error)=w182) -> (error out=w181:errorcluster)
        n50 = call <vilib>:"Clear Errors.vi"("error in (no error)"=w181) -> ()  [unwired: 5 in, 2 out]
      }
      event "Help Button": Value Change {
        n51 = event-data() -> ()  [unwired: 1 in, 6 out]
        n52 = call "Run_VI.vi"("Nome.vi"="Help_geral.vi", "Origem_VI"=enum16{"VI_esta_no_meu_PC", "VI_esta_na_rede"}."VI_esta_no_meu_PC") -> ("error out"=w194:errorcluster, "reference out"=w195:refnum<vi>)  [unwired: 8 in]
        n53 = Close Reference(reference=w195, error in (no error)=w194) -> (error out=w193:errorcluster)
        n54 = call <vilib>:"Clear Errors.vi"("error in (no error)"=w193) -> ()  [unwired: 5 in, 2 out]
      }
      event "Abre conversao e link": Value Change {
        n55 = event-data() -> ()  [unwired: 1 in, 6 out]
        n56 = invoke class="VI" method="FP.Open"(reference=w202, error in=w201, "Activate"=TRUE ("Activate?"), "State"=T10."Maximized") -> (reference out=w199:refnum<vi>, error out=w198:errorcluster)  [unwired: 1 in, 3 out]
      }
      event "[ESC]": Value Change {
        w214 = T2 {"UCM.004.EEL.0300_ENTRADA"={"DIGITAL"={"X30 1"=FALSE, "X30 2"=FALSE, "X30 3"=FALSE, "X30 4"=FALSE, "X30 5"=FALSE, "X30 6"=FALSE, "X30 7"=FALSE, "X30 8"=FALSE, "X30 9"=FALSE, "X30 10"=FALSE, "X30 11"=FALSE, "X30 12"=FALSE, "X30 13"=FALSE, "X30 14"=FALSE, "X30 15"=FALSE, "X30 16"=FALSE, "SPK-RD-ALR"=FALSE, "SPK-RD-VVT"=FALSE, "SPK-RD-FLL"=FALSE, "SPW-RD-ALR"=FALSE, "SPW-RD-VVT"=FALSE, "SPW-RD-FLL"=FALSE}, "ANALOGICO"={"SKM-PA-BAR"=0, "SKM-PA-TQ"=0, "SKM-TI-TQ"=0, "SKM-PA-LAM"=0, "SKM-TI-LAM"=0, "SKM-PD-LAM"=0, "SKM-TI-WF"=0, "SKM-FIM-WF"=0, "SIT-PI-001"=0, "SKI-PD-ST"=0, "SIT-PI-MS1"=0, "SIT-PI-MS2"=0, "SKM-TI-KF"=0, "SPW-PD-P"=0, "SPK-PD-P"=0, "X32 16 "=0, "X32 17"=0, "X32 18"=0, "X32 19"=0, "X32 20"=0, "X32 21"=0, "X32 22"=0, "X32 23"=0, "X32 24"=0, "SPK-RD-ST"=0, "SPW-RD-ST"=0, "SPK-RD-VEL"=0, "SPW-RD-VEL"=0, "SPK-RD-IA"=0, "SPW-RD-IA"=0, "SPK-RD-TU"=0, "SPW-RD-TU"=0, "SKM-TI-COR-KF"=0.0, "SKM-DEN-COR-KF"=0.0, "SKM-FIC-COR-KF"=0.0, "SKM-TI-COR-AR"=0.0, "SKM-DEN-COR-AR"=0.0, "SPK-RD-CRT"=0.0, "SPW-RD-CRT"=0.0, "SKM-FIC-COR-AR"=0.0}}, "UCM.004.EEL.0200_ENTRADA"={"DIGITAL"={"SKS-LAH-S"=FALSE, "SKS-LAH-W"=FALSE, "SKS-LAH-K"=FALSE, "SKS-MIN-W"=FALSE, "SKS-MAX-W"=FALSE, "SKS-MIN-K"=FALSE, "SKS-MAX-K"=FALSE, "X30-8"=FALSE, "X30-9"=FALSE, "X30-10"=FALSE, "X30-11"=FALSE, "X30-12"=FALSE, "X30-13"=FALSE, "X30-14"=FALSE, "X30-15"=FALSE, "X30-16"=FALSE}, "ANALOGICO"={"SKS-LC-K"=0, "SKS-LC-W"=0, "SHD-TI-AMB"=0, "X32-4"=0, "SHD-PI-01"=0, "SHD-PI-02"=0, "SIT-PI-MS3"=0, "SIT-PI-03"=0}}, "INTERNO"={"DIGITAL"={"INTERNO-SI-SS-1"=FALSE, "INTERNO-SI-SS-2"=FALSE, "INTERNO-SI-SS-3"=FALSE, "INTERNO-SS-SW-1"=FALSE, "INTERNO-SS-SK-1"=FALSE}, "ANALOGICO"={"com_pc_analog"=0.0}}}  # todos_os_dados_ENTRADA
        w215 = T6 {"UCM.004.EEL.0300_SAIDA"={"DIGITAL"={"SPK-CV-001"=FALSE, "SPK-CV-002"=FALSE, "SPK-CV-003"=FALSE, "SPK-CV-004"=FALSE, "SPK-CV-005"=FALSE, "SPK-CV-006"=FALSE, "SPK-CV-007"=FALSE, "SPK-CV-008"=FALSE, "SPW-CV-001"=FALSE, "SPW-CV-002"=FALSE, "SPW-CV-003"=FALSE, "SPW-CV-004"=FALSE, "SPW-CV-005"=FALSE, "SPW-CV-006"=FALSE, "SPW-CV-007"=FALSE, "SPW-CV-008"=FALSE, "SKM-CV-LAM"=FALSE, "SKM-CV-COR"=FALSE, "SKM-CV-JMP"=FALSE, "SKI-CV-AR"=FALSE, "SKI-CV-KF-ST"=FALSE, "SKI-CV-KF-BY1"=FALSE, "SKI-CV-WF-ST"=FALSE, "SKI-CV-WF-BY1"=FALSE, "SKI-CV-ST"=FALSE, "SKI-CV-BY2"=FALSE, "X31-27"=FALSE, "X31-28"=FALSE, "X31-29"=FALSE, "X31-30"=FALSE, "X31-31"=FALSE, "X31-32"=FALSE, "PID-PC-TQ-ON"=FALSE, "PID-FC-AR-ON"=FALSE, "PID-WF-ON"=FALSE, "PID-KF-ON"=FALSE, "PID-SA-WF-INV"=FALSE, "PID-SA-KF-INV"=FALSE, "PID-SA-AR-COR"=FALSE, "SPK-WR-ON"=FALSE, "SPW-WR-ON"=FALSE, "SPK-WR-OFF"=FALSE, "SPW-WR-OFF"=FALSE}, "ANALOGICO"={"SKM-PC-TQ"=0, "SKM-FC-AR"=0, "SKM-FC-WF"=0, "SKM-FC-KF"=0, "X33 5"=0, "X33 6"=0, "X33 7"=0, "X33 8"=0, "X33 9"=0, "X33 10"=0, "X33 11"=0, "X33 12"=0, "X33 13"=0, "X33 14"=0, "PID-PC-TQ-SP"=0, "PID-FC-AR-SP"=0, "PID-FC-WF-SP"=0, "PID-FC-KF-SP"=0, "PID-INC-WF-SP"=0, "PID-INC-KF-SP"=0, "SPK-WR-VEL"=0, "SPW-WR-VEL"=0, "SKM-FIC-COR-AR-MAX"=0.0, "SKM-FIC-COR-AR-MIN"=0.0, "SKM-FIC-COR-KF-MAX"=0.0, "SKM-FIC-COR-KF-MIN"=0.0, "PID-PC-TQ-GP"=0.0, "PID-PC-TQ-GI"=0.0, "PID-PC-TQ-GD"=0.0, "PID-FC-AR-GP"=0.0, "PID-FC-AR-GI"=0.0, "PID-FC-AR-GD"=0.0, "PID-FC-WF-GP"=0.0, "PID-FC-WF-GI"=0.0, "PID-FC-WF-GD"=0.0, "PID-FC-KF-GP"=0.0, "PID-FC-KF-GI"=0.0, "PID-FC-KF-GD"=0.0, "PID-INV-WF-GP"=0.0, "PID-INV-WF-GI"=0.0, "PID-INV-WF-GD"=0.0, "PID-INV-KF-GP"=0.0, "PID-INV-KF-GI"=0.0, "PID-INV-KF-GD"=0.0}}, "UCM.004.EEL.0200_SAIDA"={"DIGITAL"={"SKS-CV-001"=FALSE, "SKS-CV-002"=FALSE, "SKS-CV-003"=FALSE, "SKS-CV-004"=FALSE, "SKS-CV-005"=FALSE, "SKS-CV-006"=FALSE, "SHD-CV-001"=FALSE, "SHD-CV-002"=FALSE, "SHD-ON-OFF"=FALSE, "X31-10"=FALSE, "X31-11"=FALSE, "X31-12"=FALSE, "X31-13"=FALSE, "X31-14"=FALSE, "X31-15"=FALSE, "X31-16"=FALSE}, "ANALOGICO"={"GD-ST-ES"=0, "X33-2"=0}}, "INTERNO"={"DIGITAL"={"INTERNO-SI-SS-1"=FALSE, "INTERNO-SI-SS-2"=FALSE, "INTERNO-SI-SS-3"=FALSE, "INTERNO-SS-SW-1"=FALSE, "INTERNO-SS-SK-1"=FALSE}, "ANALOGICO"={"com_pc_analog"=0.0}}}  # todos_os_dados_SAIDA
        n57 = event-data() -> ()  [unwired: 1 in, 6 out]
        n58 = for {
          tunnel: w228 -> [w233]
          tunnel: w219 -> [w232] mode=indexing
          n59 = TCP Close Connection(connection ID=w232, error in (no error)=w233) -> (error out=w231:errorcluster)  [unwired: 1 in, 1 out]
          n60 = call <vilib>:"Clear Errors.vi"("error in (no error)"=w231) -> ()  [unwired: 5 in, 2 out]
        }
        n61 = invoke class="VI" method="Ctrl Val.Set"(reference=w225, error in=w224, "Control Name"="[ESC]", "Value"=TRUE) -> (reference out=w221:refnum<vi>, error out=w220:errorcluster)  [unwired: 1 in, 3 out]
        n62 = case shown="Error .." w228 {
          selector: w228 -> [w234 w236]
          tunnel: [w234 w235] -> w229
          frame No Error {
          }
          frame Error {
            n63 = call <vilib>:"Clear Errors.vi"("error in (no error)"=w236) -> ("error out"=w235:errorcluster)  [unwired: 5 in, 1 out]
          }
        }
        n64 = invoke class="VI" method="Ctrl Val.Set"(reference=w211, error in=w210, "Control Name"="stop", "Value"=TRUE) -> (reference out=w209:refnum<vi>, error out=w208:errorcluster)  [unwired: 1 in, 3 out]
        n65 = local write "Quantidade de Clients"(0 ("Quantidade de Clients")) -> ()
        n66 = local write "Clients Conectados"(string[] [] ("Clients Conectados")) -> ()
        n67 = local write "led_indica_server_ligado"(FALSE ("Boolean")) -> ()
        n68 = local write "engenharia_todos_os_dados_ENTRADA"(w214) -> ()
        n69 = local write "status"("VI encontra-se desligada:\nAperte Ctrl+R caso deseje rodar") -> ()
        n70 = local write "IPs Conectados"(string[] [] ("IPs Conectados")) -> ()
        n71 = local write "todos_dados_SAIDA"(w215) -> ()
      }
    }
  }
  n72 = call <vilib>:"Clear Errors.vi"("error in (no error)"=w13) -> ()  [unwired: 5 in, 2 out]
  n73 = invoke class="VI" method="Abort VI"(reference=w19, error in=w18) -> (reference out=w17:refnum<vi>, error out=w16:errorcluster)  [unwired: 1 in, 1 out]
  n74 = invoke class="VI" method="FP.Close"(reference=w4, error in=w3) -> (reference out=w2:refnum<vi>, error out=w1:errorcluster)  [unwired: 1 in, 1 out]
  n75 = Close Reference(reference=w17, error in (no error)=w16) -> (error out=w15:errorcluster)
  n76 = invoke class="VI" method="Abort VI"(reference=w2, error in=w1) -> (reference out=w5:refnum<vi>, error out=w6:errorcluster)  [unwired: 1 in, 1 out]
  n77 = call <vilib>:"Clear Errors.vi"("error in (no error)"=w15) -> ()  [unwired: 5 in, 2 out]
  n78 = Close Reference(reference=w5, error in (no error)=w6) -> (error out=w7:errorcluster)
  n79 = call <vilib>:"Clear Errors.vi"("error in (no error)"=w7) -> ()  [unwired: 5 in, 2 out]
